vi "verify connector pane.vi"(9 "Control pane terminals":T1(array[cluster]), 11 "VI":refnum<vi>) -> (2 "VI fits specs?":bool)   [LabVIEW 2009]
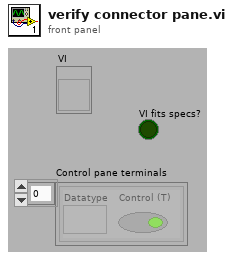
[diagram p1: front panel]
types:
  T1 = cluster{"Datatype":variant, "Control (T)":bool}[]
  T2 = typedef "datatype.ctl" = enum8{"<Null>", "Cluster", "Array", "Boolean", "Path", "String", "Number", "Refnum", "Waveform", "Pict", "DAQ"}
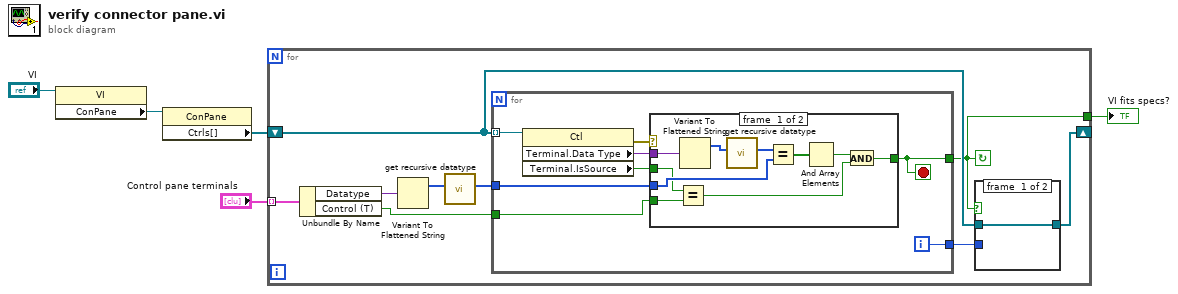
[diagram p0: block diagram]
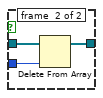
[diagram p2: hidden frame]
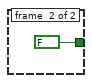
[diagram p3: hidden frame]
diagram:
  n1 = property class="VI"(reference="VI") -> ("ConPane"=w5:refnum<vi>)  [unwired: 1 in, 2 out]
  n2 = property class="ConPane"(reference=w5) -> ("Ctrls[]"=w4:refnum<vi>[])  [unwired: 1 in, 2 out]
  n3 = for {
    tunnel: "Control pane terminals" -> [w14] mode=indexing
    shift-right: [w9] -> _
    shift-left: w4 -> [w10]
    tunnel: [w8] -> w1
    stop <- w8 continue-if-true
    n4 = Unbundle By Name(w14) -> ("Datatype"=w13:variant, "Control (T)"=w12:bool)
    n5 = Variant To Flattened String(Variant=w13) -> (1:w7:i16[])  [unwired: 1 out]
    n6 = call "get recursive datatype.vi"("Type Descriptor"=w7) -> ("Recursive Datatype"=w6:T2[])  [unwired: 9 in, 1 out]
    n7 = for {
      tunnel: w10 -> [w26] mode=indexing
      tunnel: w6 -> [w24]
      tunnel: w12 -> [w22]
      tunnel: [w21] -> w8
      tunnel: [w20] -> w11
      i -> [w20]
      stop <- w21 stop-if-true
      n8 = property class="Ctl"(reference=w26) -> (error out=w19:errorcluster, "Terminal.Data Type"=w25:variant, "Terminal.IsSource"=w23:bool)  [unwired: 1 in, 1 out]
      n9 = case shown="No Error" w19 {
        tunnel: w25 -> [w36 _]
        tunnel: w24 -> [w35 _]
        tunnel: w23 -> [w34 _]
        tunnel: w22 -> [w33 _]
        tunnel: [w29 FALSE] -> w21
        frame #0 {
          n10 = Equal?(x=w34, y=w33) -> (x = y?=w30:bool)
          n11 = Variant To Flattened String(Variant=w36) -> (1:w28:i16[])  [unwired: 1 out]
          n12 = call "get recursive datatype.vi"("Type Descriptor"=w28) -> ("Recursive Datatype"=w27:T2[])  [unwired: 9 in, 1 out]
          n13 = Equal?(x=w27, y=w35) -> (x = y?=w32:bool[])
          n14 = And Array Elements(Boolean array=w32) -> (logical AND=w31:bool)
          n15 = And(x=w31, y=w30) -> (x .and. y?=w29:bool)
        }
        frame #1 {
        }
      }
    }
    n16 = case shown="True" w8 {
      tunnel: w11 -> [_ w16]
      tunnel: w10 -> [w15 w18]
      tunnel: [w15 w17] -> w9
      frame #0 {
      }
      frame #1 {
        n17 = Delete From Array(array=w18, index=w16) -> (array with subset deleted=w17:refnum<vi>[])  [unwired: 1 in, 1 out]
      }
    }
  }
  "VI fits specs?" <- w1
